vi "Save Peak data.vi"(0 "Min Cluster":T2 {"Hour" format="%<%H:%M>t"}, 4 "Max cluster":T1 {"Hour" format="%<%H:%M>t"}, 5 "file path (use dialog)":path, 6 "Average profile":dbl[](array[numeric]) format="%.2f", 7 "Days":string, 8 "Average Demand / day":dbl format="%.2f", 9 "Total demand":dbl format="%.2f", 10 "%":dbl[](array[numeric]) format="%.2f", 11 "Strings []":string[](array[string])) -> (3 "path":path)   [LabVIEW 2018]
panel:
  out "resulting string":string
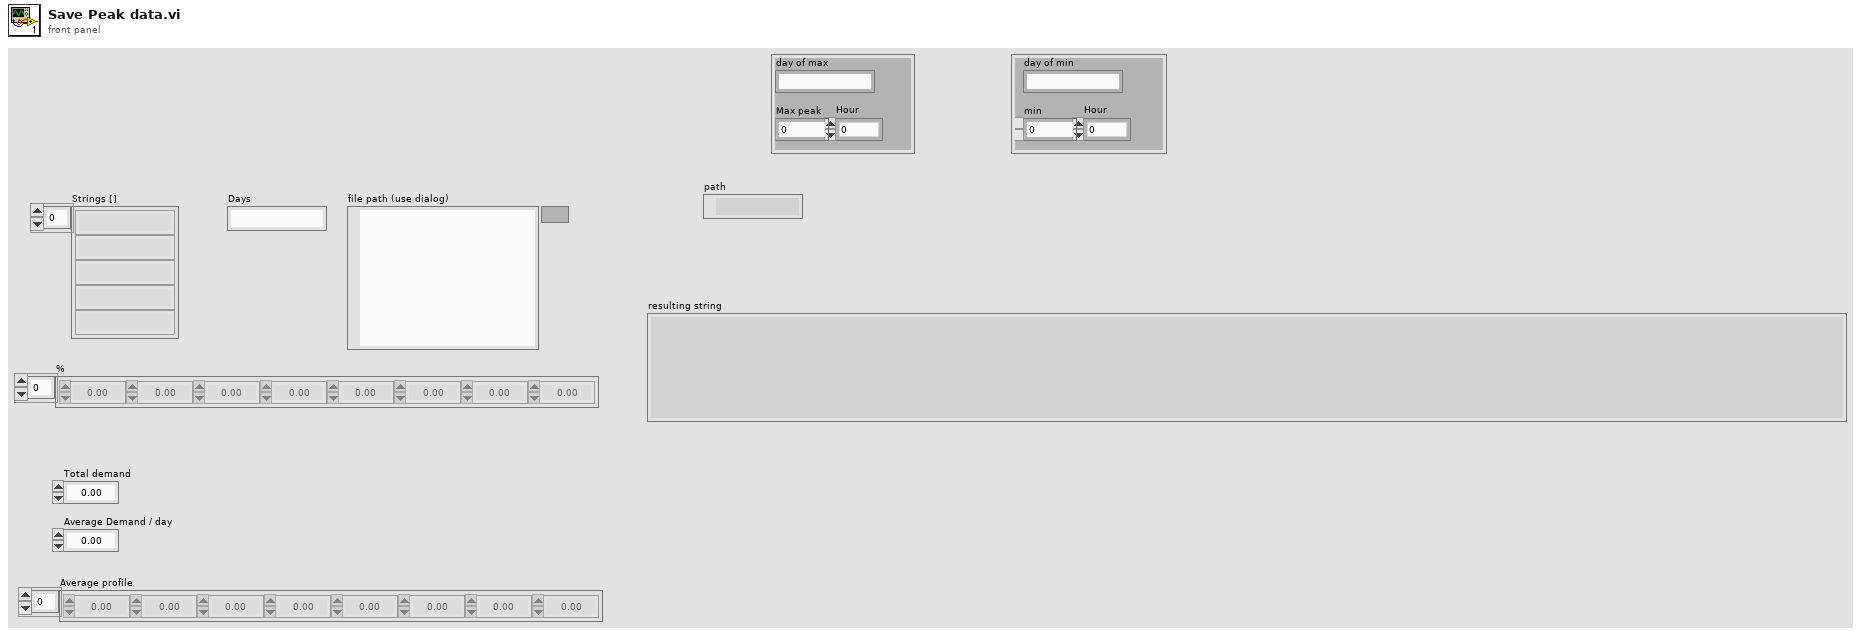
[diagram p1: front panel]
types:
  T1 = cluster{"Hour":i32, "Max peak":dbl, "day of max":string}
  T2 = cluster{"Hour":i32, "min":dbl, "day of min":string}
  T3 = enum16{"open", "replace", "create", "open or create", "replace or create", "replace or create with confirmation"}
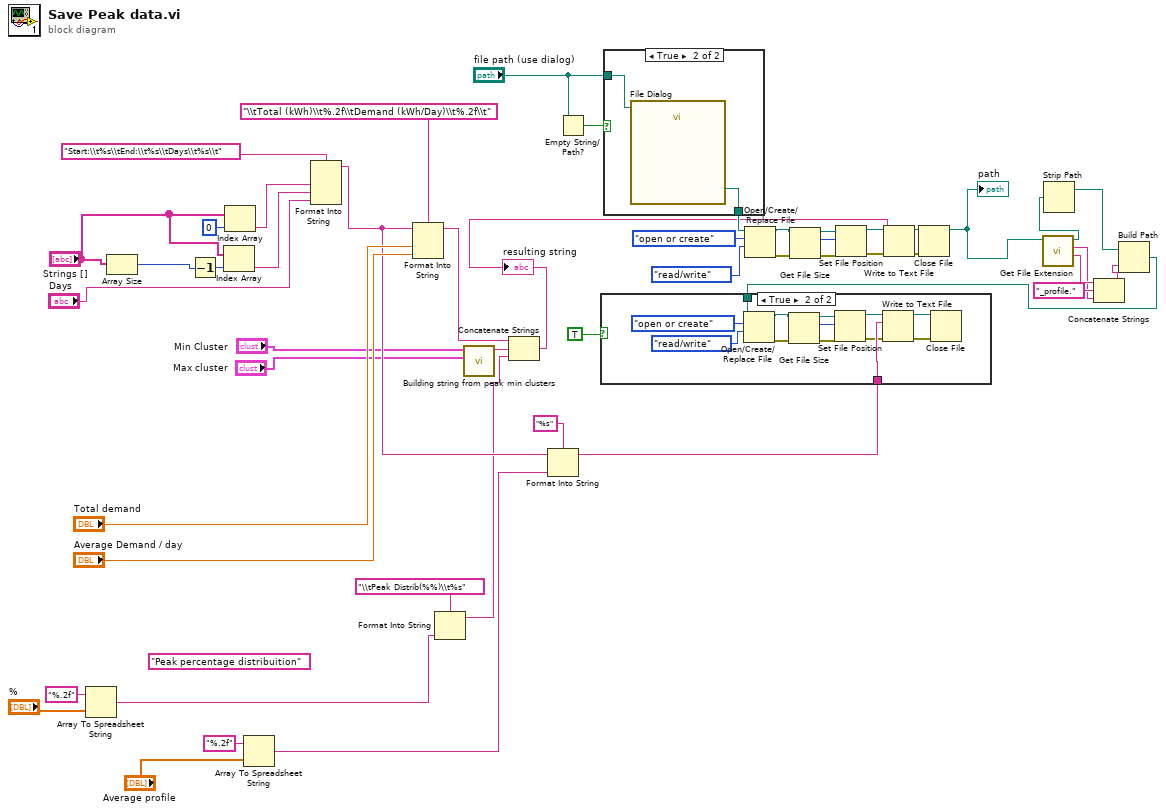
[diagram p0: block diagram]
diagram:
  (unwired) "Peak percentage distribuition" ("format string")
  n1 = Array To Spreadsheet String(array="%", 3:"%.2f" ("format string")) -> (spreadsheet string=w2:string)  [unwired: 1 in]
  n2 = Array Size(array="Strings []") -> (size(s)=w49:i32)
  n3 = Decrement(x=w49) -> (x-1=w48:i32)
  n4 = Index Array(array="Strings []", index=w48) -> (element=w35:string)
  n5 = Index Array(array="Strings []", index=0) -> (element=w36:string)
  n6 = Array To Spreadsheet String(array="Average profile", 3:"%.2f" ("format string")) -> (spreadsheet string=w39:string)  [unwired: 1 in]
  n7 = Format Into String(format string="Start:\\t%s\\tEnd:\\t%s\\tDays\\t%s\\t", w36, w35, "Days") -> (resulting string=w34:string)  [unwired: 2 in, 1 out]
  n8 = Format Into String(format string="\\tTotal (kWh)\\t%.2f\\tDemand (kWh/Day)\\t%.2f\\t", initial string=w34, "Total demand", "Average Demand / day") -> (resulting string=w5:string)  [unwired: 1 in, 1 out]
  n9 = Format Into String(format string="\\tPeak Distrib(%%)\\t%s", w2) -> (resulting string=w1:string)  [unwired: 2 in, 1 out]
  n10 = call "Building string from peak min clusters.vi"("Max cluster"="Max cluster", "Min Cluster"="Min Cluster") -> ("resulting string 2"=w7:string)  [unwired: 9 in]
  n11 = Concatenate Strings(w5, w7, w1) -> (w4:string)
  "resulting string" <- w4
  n12 = Format Into String(format string="%s", initial string=w34, w39) -> (resulting string=w6:string)  [unwired: 1 in, 1 out]
  n13 = Empty String/Path?(string/path="file path (use dialog)") -> (empty?=w12:bool)
  n14 = case shown="True" w12 {
    tunnel: "file path (use dialog)" -> [w51 w53]
    tunnel: [w51 w52] -> w14
    frame False {
    }
    frame True {
      n15 = call "File Dialog"("start path"=w53) -> ("selected path"=w52:path)  [unwired: 11 in, 3 out]
    }
  }
  n16 = Open/Create/Replace File(file path (use dialog)=w14, operation (0:open)=T3."open or create", access (0:read/write)=enum16{"read/write", "read-only", "write-only"}."read/write") -> (refnum out=w25:refnum<file>, error out=w23:errorcluster)  [unwired: 3 in, 1 out]
  n17 = Get File Size(file=w25, error in=w23) -> (refnum out=w26:refnum<file>, size (in bytes)=w27:i64, 0:w28:errorcluster)
  n18 = Set File Position(offset (in bytes) (0)=w27, refnum=w26, error in=w28) -> (refnum out=w24:refnum<file>, error out=w22:errorcluster)  [unwired: 1 in]
  n19 = Write to Text File(file (use dialog)=w24, text=w4, error in=w22) -> (refnum out=w32:refnum<file>, error out=w31:errorcluster)  [unwired: 1 in, 1 out]
  n20 = Close File(refnum=w32, error in=w31) -> (path=w11:path)  [unwired: 1 out]
  "path" <- w11
  n21 = call <vilib>:"Get File Extension.vi"("file"=w11) -> ("filename without extension"=w21:string, "lowercase file extension"=w19:string, "dup file"=w16:path)  [unwired: 6 in, 2 out]
  n22 = Strip Path(path=w16) -> (stripped path=w15:path)  [unwired: 1 out]
  n23 = Concatenate Strings(w21, "_profile." ("string"), w19) -> (w18:string)
  n24 = Build Path(base path=w15, name or relative path=w18) -> (appended path=w17:path)
  n25 = case shown="True" TRUE {
    tunnel: w6 -> [_ w66]
    tunnel: w17 -> [_ w55]
    frame False {
    }
    frame True {
      n26 = Open/Create/Replace File(file path (use dialog)=w55, operation (0:open)=T3."open or create", access (0:read/write)=enum16{"read/write", "read-only", "write-only"}."read/write") -> (refnum out=w62:refnum<file>, error out=w64:errorcluster)  [unwired: 3 in, 1 out]
      n27 = Get File Size(file=w62, error in=w64) -> (refnum out=w61:refnum<file>, size (in bytes)=w60:i64, 0:w59:errorcluster)
      n28 = Set File Position(offset (in bytes) (0)=w60, refnum=w61, error in=w59) -> (refnum out=w63:refnum<file>, error out=w65:errorcluster)  [unwired: 1 in]
      n29 = Write to Text File(file (use dialog)=w63, text=w66, error in=w65) -> (refnum out=w56:refnum<file>, error out=w57:errorcluster)  [unwired: 1 in, 1 out]
      n30 = Close File(refnum=w56, error in=w57) -> ()  [unwired: 2 out]
    }
  }
